vi "notify parent.vi"(7 "enqueue setting":T1, 8 "error in":errorcluster, 9 "timeout in ms (-1)":i32=-1, 10 "element":refnum<class "communicator message.lvclass">, 11 "communicator in":refnum<class "communicator.lvclass">) -> (0 "error out":errorcluster)   [LabVIEW 2015, in "communicator.lvclass"]
uses:
  communicator.lvclass
  message/communicator message.lvclass
  communicator queue/enqueue variety.ctl
  communicator.lvclass/communicator.ctl
  communicator queue/identifying queue.lvclass/identifying queue.ctl
  message/set sender.vi
  communicator queue/identifying queue.lvclass
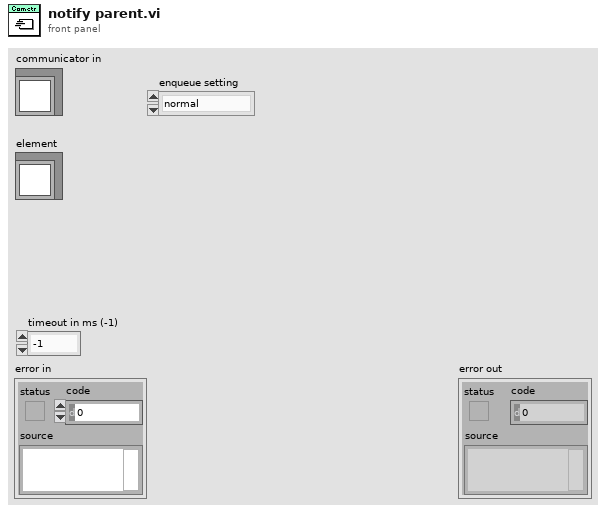
[diagram p1: front panel]
types:
  T1 = typedef "identifying queue.lvclass/enqueue variety.ctl" = enum16{"normal", "lossy", "priority"}
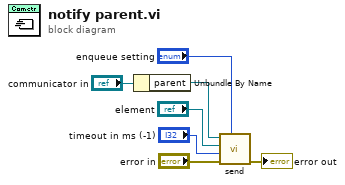
[diagram p0: block diagram]
diagram:
  n1 = Unbundle By Name("communicator in") -> ("parent"=w6:refnum<class "identifying queue.lvclass">)
  n2 = call "send.vi"("enqueue command"="enqueue setting", "error in"="error in", "timeout in ms (-1)"="timeout in ms (-1)", "message"="element", "message connection in"=w6) -> ("error out"=→"error out":errorcluster)  [unwired: 5 in, 1 out]
